vi "COMM.vi"() -> ()   [LabVIEW 2018]
uses:
  socket PUB/socket PUB.lvclass
  C:/Users/Denis/Desktop/FWCS/FWCS/ECP/Socket/Socket.lvclass
  socket SUB/socket SUB.lvclass
  RxTx/CM_RxTx.lvclass
  Socket/Socket.lvclass
  <vilib>/addons/zeromq/zmq_context.lvclass
panel:
  in  "log file path":path=path "C:/Users/Denis/Desktop/FWCS/FWCS/ECP/CFG file"
  out "error out 3":errorcluster
  in  "socket SUB.lvclass":refnum<class "socket SUB.lvclass">
  in  "socket PUB.lvclass":refnum<class "socket PUB.lvclass">
  # "PUB endpoint"
  # "SUB endpoint"
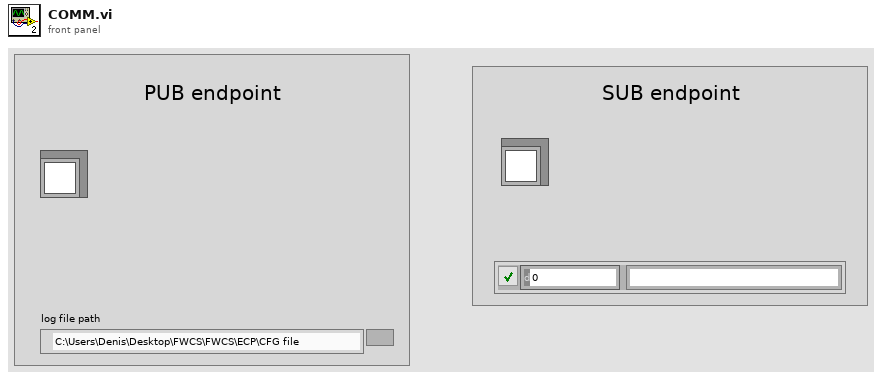
[diagram p1: front panel]
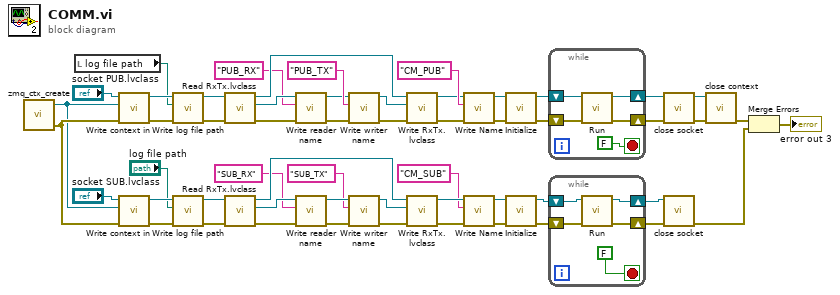
[diagram p0: block diagram]
diagram:
  n1 = call <vilib>:"zmq_ctx_create.vi"() -> ("error out"=w19:errorcluster, "context out"=w18:refnum<class "zmq_context.lvclass">)  [unwired: 4 in]
  n2 = local read "log file path"() -> (w2:path)
  n3 = call-dynamic "Write context in.vi"("error in (no error)"=w19, "zeromq.lvlib:ZeroMQ Context"=w18, "Socket in"="socket PUB.lvclass") -> ("error out"=w8:errorcluster, "Socket out"=w11:refnum<class "socket PUB.lvclass">)  [unwired: 7 in]
  n4 = call-dynamic "Write context in.vi"("error in (no error)"=w19, "zeromq.lvlib:ZeroMQ Context"=w18, "Socket in"="socket SUB.lvclass") -> ("error out"=w7:errorcluster, "Socket out"=w4:refnum<class "socket SUB.lvclass">)  [unwired: 7 in]
  n5 = call-dynamic "Write log file path.vi"("error in (no error)"=w8, "log file path"=w2, "Socket in"=w11) -> ("error out"=w9:errorcluster, "Socket out"=w10:refnum<class "socket PUB.lvclass">)  [unwired: 7 in]
  n6 = call-dynamic "Write log file path.vi"("error in (no error)"=w7, "log file path"="log file path", "Socket in"=w4) -> ("error out"=w5:errorcluster, "Socket out"=w6:refnum<class "socket SUB.lvclass">)  [unwired: 7 in]
  n7 = call-dynamic "Read RxTx.lvclass.vi"("error in (no error)"=w9, "Socket in"=w10) -> ("error out"=w48:errorcluster, "RxTx.lvclass"=w52:refnum<class "CM_RxTx.lvclass">, "Socket out"=w49:refnum<class "socket PUB.lvclass">)  [unwired: 7 in]
  n8 = call-dynamic "Read RxTx.lvclass.vi"("error in (no error)"=w5, "Socket in"=w6) -> ("error out"=w29:errorcluster, "RxTx.lvclass"=w25:refnum<class "CM_RxTx.lvclass">, "Socket out"=w28:refnum<class "socket SUB.lvclass">)  [unwired: 7 in]
  n9 = call-dynamic "Write reader name.vi"("error in (no error)"=w48, "RX name"="PUB_RX" ("reader name"), "RxTx in"=w52) -> ("error out"=w47:errorcluster, "RxTx out"=w51:refnum<class "CM_RxTx.lvclass">)  [unwired: 7 in]
  n10 = call-dynamic "Write reader name.vi"("error in (no error)"=w29, "RX name"="SUB_RX" ("reader name"), "RxTx in"=w25) -> ("error out"=w30:errorcluster, "RxTx out"=w26:refnum<class "CM_RxTx.lvclass">)  [unwired: 7 in]
  n11 = call-dynamic "Write writer name.vi"("error in (no error)"=w47, "Tx name"="PUB_TX" ("writer name"), "RxTx in"=w51) -> ("error out"=w46:errorcluster, "RxTx out"=w50:refnum<class "CM_RxTx.lvclass">)  [unwired: 7 in]
  n12 = call-dynamic "Write writer name.vi"("error in (no error)"=w30, "Tx name"="SUB_TX" ("writer name"), "RxTx in"=w26) -> ("error out"=w31:errorcluster, "RxTx out"=w27:refnum<class "CM_RxTx.lvclass">)  [unwired: 7 in]
  n13 = call-dynamic "Write RxTx.lvclass.vi"("error in (no error)"=w46, "RxTx.lvclass"=w50, "Socket in"=w49) -> ("error out"=w36:errorcluster, "Socket out"=w37:refnum<class "socket PUB.lvclass">)  [unwired: 7 in]
  n14 = call-dynamic "Write RxTx.lvclass.vi"("error in (no error)"=w31, "RxTx.lvclass"=w27, "Socket in"=w28) -> ("error out"=w34:errorcluster, "Socket out"=w33:refnum<class "socket SUB.lvclass">)  [unwired: 7 in]
  n15 = call-dynamic "Write Name.vi"("error in (no error)"=w36, "Name"="CM_PUB", "Socket in"=w37) -> ("error out"=w44:errorcluster, "Socket out"=w45:refnum<class "socket PUB.lvclass">)  [unwired: 7 in]
  n16 = call-dynamic "Write Name.vi"("error in (no error)"=w34, "Name"="CM_SUB", "Socket in"=w33) -> ("error out"=w20:errorcluster, "Socket out"=w21:refnum<class "socket SUB.lvclass">)  [unwired: 7 in]
  n17 = call-dynamic "Initialize.vi"("error in (no error)"=w44, "socket PUB in"=w45) -> ("error out"=w41:errorcluster, "socket PUB out"=w43:refnum<class "socket PUB.lvclass">)  [unwired: 8 in]
  n18 = call-dynamic "Initialize.vi"("error in (no error)"=w20, "socket SUB in"=w21) -> ("error out"=w16:errorcluster, "socket SUB out"=w17:refnum<class "socket SUB.lvclass">)  [unwired: 8 in]
  n19 = while {
    shift-right: [w58] -> w42
    shift-left: w43 -> [w60]
    shift-right: [w57] -> w40
    shift-left: w41 -> [w59]
    stop <- FALSE stop-if-true
    n20 = call-dynamic "Run.vi"("error in (no error)"=w59, "socket PUB in"=w60) -> ("error out"=w57:errorcluster, "socket PUB out"=w58:refnum<class "socket PUB.lvclass">)  [unwired: 8 in]
  }
  n21 = while {
    shift-right: [w63] -> w14
    shift-left: w17 -> [w65]
    shift-right: [w62] -> w15
    shift-left: w16 -> [w64]
    stop <- FALSE stop-if-true
    n22 = call-dynamic "Run.vi"("error in (no error)"=w64, "socket SUB in"=w65) -> ("error out"=w62:errorcluster, "socket SUB out"=w63:refnum<class "socket SUB.lvclass">)  [unwired: 8 in]
  }
  n23 = call "close socket.vi"("error in (no error)"=w40, "Socket in"=w42) -> ("error out"=w55:errorcluster, "Socket out"=w54:refnum<class "socket PUB.lvclass">)  [unwired: 8 in]
  n24 = call "close socket.vi"("error in (no error)"=w15, "Socket in"=w14) -> ("error out"=w13:errorcluster)  [unwired: 8 in, 1 out]
  n25 = call-dynamic "close context.vi"("error in (no error)"=w55, "Socket in"=w54) -> ("error out"=w1:errorcluster)  [unwired: 8 in, 1 out]
  n26 = Merge Errors(w1, w13) -> (→"error out 3":errorcluster)
